vi "Get_Percentage_of_Amp.vi"(0 "Amplitude(V)":dbl=5.0, 5 "End_Point_Per (70%)":dbl=0.7 format="%#_13g", 7 "Start_Point_Per (30%)":dbl=0.3 format="%#_13g", 9 "Min (0%)":dbl format="%#_13g") -> (4 "End_Point":dbl, 6 "Start_Point":dbl, 8 "Min_Point":dbl)   [LabVIEW 2023]
doc: "This VI gives the End point, start point and min point when amplitude is given in."
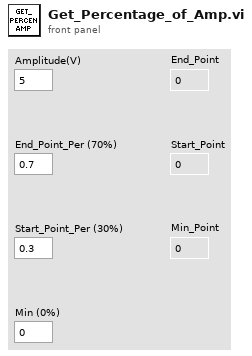
[diagram p1: front panel]
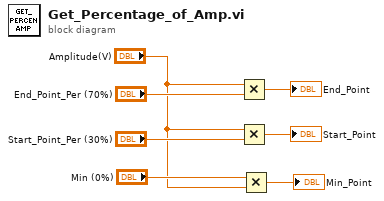
[diagram p0: block diagram]
diagram:
  n1 = Multiply(x="Amplitude(V)", y="End_Point_Per (70%)") -> (x*y=→"End_Point":dbl)
  n2 = Multiply(x="Amplitude(V)", y="Start_Point_Per (30%)") -> (x*y=→"Start_Point":dbl)
  n3 = Multiply(x="Min (0%)", y="Amplitude(V)") -> (x*y=→"Min_Point":dbl)
